vi "Instrument.OxfordVRM.Get All.vi"(8 "error in (no error)":errorcluster, 11 "Instrument.OxfordVRM in":refnum<class "Instrument.OxfordVRM.lvclass">) -> (0 "error out":errorcluster, 2 "getAll":T1, 3 "Instrument.OxfordVRM out":refnum<class "Instrument.OxfordVRM.lvclass">)   [LabVIEW 2019, in "Instrument.OxfordVRM.lvclass"]
uses:
  Instrument.OxfordVRM.lvclass
  51bec6ce-7eba-4b7b-b77e-ed0eea84607f.vi
  Typedefs/getAll.ctl
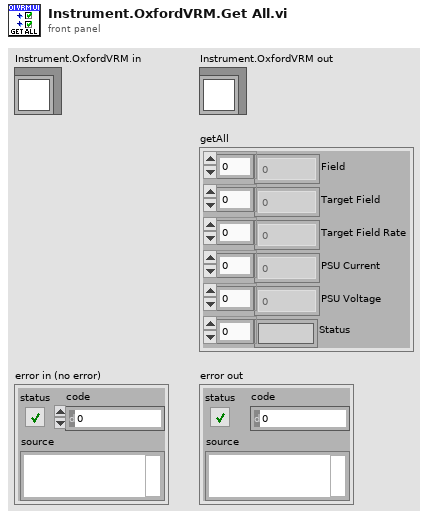
[diagram p1: front panel]
types:
  T1 = typedef "Instrument.OxfordVRM.lvclass/getAll.ctl" = cluster{"Field":dbl[], "Target Field":dbl[], "Target Field Rate":dbl[], "PSU Current":dbl[], "PSU Voltage":dbl[], "Status":string[]}
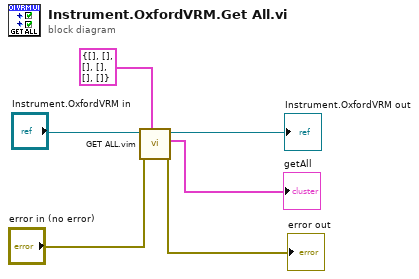
[diagram p0: block diagram]
diagram:
  n1 = call "GET ALL.vim"("type"=T1 {"Field"=[], "Target Field"=[], "Target Field Rate"=[], "PSU Current"=[], "PSU Voltage"=[], "Status"=[]} ("getAll"), "error in (no error)"="error in (no error)", "Instrument in"="Instrument.OxfordVRM in") -> ("error out"=→"error out":errorcluster, "getAll"=→"getAll":T1, "Instrument out"=→"Instrument.OxfordVRM out":refnum<class "Instrument.OxfordVRM.lvclass">)  [unwired: 6 in]
